vi "Result.Parse Exec Rtn Data, STD OUT is code, Stderr is desc, Create Result Data_V1.vi"(7 "Name":string, 8 "BaseCode":i32, 9 "RtnCode":i32, 10 "StdErr":string, 11 "StdOut":string) -> (3 "Meas":T1[](array[typedef]) {"Status" items=["LOG", "PASS", "FAIL", "ERROR"]})   [LabVIEW 2024]
uses:
  Result.Measurement Item.ctl
  Result.Measurement and Attribute Item Status.ctl
  <vilib>/Utility/error.llb/Trim Whitespace One-Sided.vi
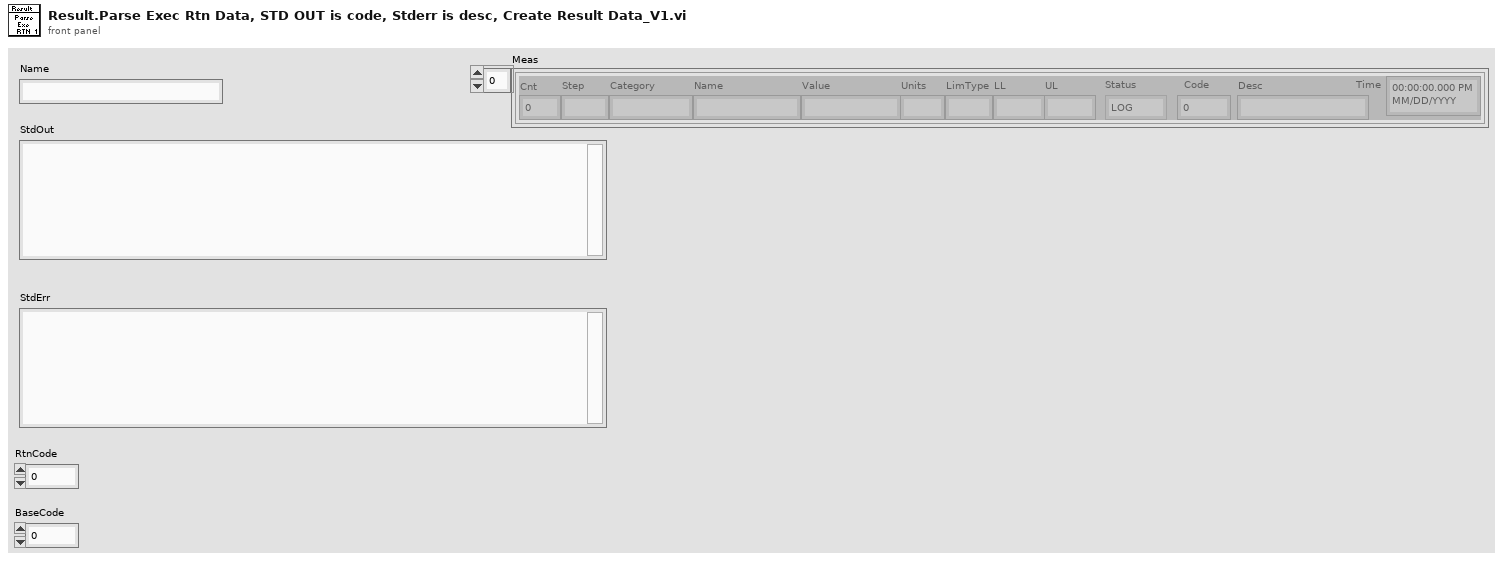
[diagram p1: front panel]
types:
  T1 = typedef "Result.Measurement Item.ctl" = cluster{"Cnt":i32, "Step":string, "Category":string, "Name":string, "Value":string, "Units":string, "LimType":string, "LL":string, "UL":string, "Status":T2, "Code":i32, "Desc":string, "Time":timestamp}
  T2 = typedef "Result.Measurement and Attribute Item Status.ctl" = i32
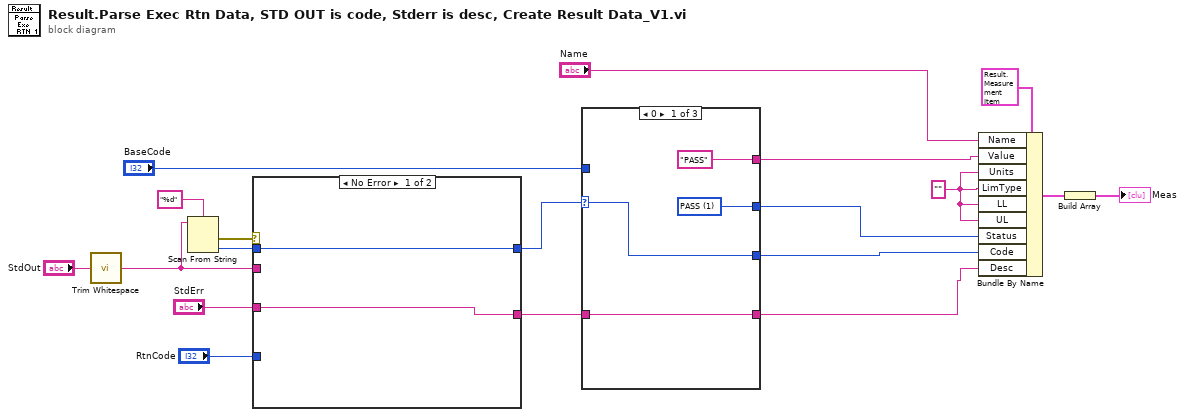
[diagram p0: block diagram]
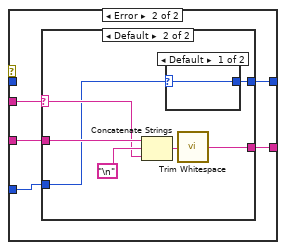
[diagram p2: hidden frame]
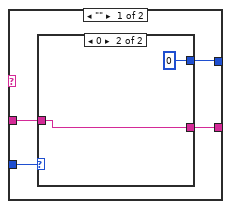
[diagram p3: hidden frame]
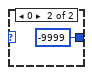
[diagram p5: hidden frame]
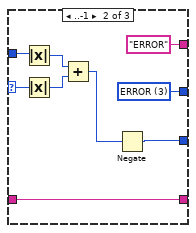
[diagram p6: hidden frame]
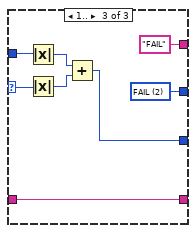
[diagram p7: hidden frame]
diagram:
  w14 = ""
  n1 = call <vilib>:"Trim Whitespace.vi"("string"="StdOut") -> ("trimmed string"=w5:string)  [unwired: 1 in]
  n2 = Scan From String(format string="%d", input string=w5) -> (error out=w8:errorcluster, output 1=w7:i32)  [unwired: 3 in, 2 out]
  n3 = case shown="No Error" w8 {
    tunnel: w7 -> [w21 _]
    tunnel: [w21 w26] -> w6
    tunnel: w5 -> [_ w24]
    tunnel: "StdErr" -> [w20 w25]
    tunnel: [w20 w23] -> w3
    tunnel: "RtnCode" -> [_ w22]
    frame No Error {
    }
    frame Error {
      n4 = case shown="Default" w24 {
        selector: w24 -> [_ w38]
        tunnel: [w29 w41] -> w26
        tunnel: w25 -> [w28 w39]
        tunnel: [w27 w36] -> w23
        tunnel: w22 -> [w30 w35]
        frame "" {
          n5 = case shown="0" w30 {
            selector: w30 -> [w32 _]
            tunnel: [w32 0] -> w29
            tunnel: w28 -> [w31 w33]
            tunnel: [w31 w33] -> w27
            frame Default {
            }
            frame 0 {
            }
          }
        }
        frame Default {
          n6 = Concatenate Strings(w39, "\n", w38) -> (w37:string)
          n7 = case shown="Default" w35 {
            selector: w35 -> [w42 _]
            tunnel: [w42 -9999] -> w41
            frame Default {
            }
            frame 0 {
            }
          }
          n8 = call <vilib>:"Trim Whitespace.vi"("string"=w37) -> ("trimmed string"=w36:string)  [unwired: 1 in]
        }
      }
    }
  }
  n9 = case shown="0" w6 {
    selector: w6 -> [w45 w54 w59]
    tunnel: [w47 w56 w64] -> w15
    tunnel: ["PASS" "ERROR" "FAIL"] -> w13
    tunnel: "BaseCode" -> [_ w53 w60]
    tunnel: [w45 w49 w58] -> w11
    tunnel: w3 -> [w44 w48 w57]
    tunnel: [w44 w48 w57] -> w2
    frame 0 {
      w47 = T2 1 items=["LOG", "PASS", "FAIL", "ERROR"] ("Status")
    }
    frame ..-1 {
      w56 = T2 3 items=["LOG", "PASS", "FAIL", "ERROR"] ("Status")
      n10 = Absolute Value(x=w53) -> (abs(x)=w52:i32)
      n11 = Absolute Value(x=w54) -> (abs(x)=w51:i32)
      n12 = Add(x=w52, y=w51) -> (x+y=w50:i32)
      n13 = Negate(x=w50) -> (-x=w49:i32)
    }
    frame 1.. {
      w64 = T2 2 items=["LOG", "PASS", "FAIL", "ERROR"] ("Status")
      n14 = Absolute Value(x=w60) -> (abs(x)=w62:i32)
      n15 = Absolute Value(x=w59) -> (abs(x)=w61:i32)
      n16 = Add(x=w62, y=w61) -> (x+y=w58:i32)
    }
  }
  n17 = Bundle By Name(cluster=T1 {"Cnt"=0, "Step"="", "Category"="", "Name"="", "Value"="", "Units"="", "LimType"="", "LL"="", "UL"="", "Status"=0, "Code"=0, "Desc"="", "Time"=timestamp(0 s since 1904-01-01)} ("Meas"), "Name"="Name", "Value"=w13, "Units"=w14, "LimType"=w14, "LL"=w14, "UL"=w14, "Status"=w15, "Code"=w11, "Desc"=w2) -> (w18:T1)
  n18 = Build Array(w18) -> (→"Meas":T1[])
